vi "Replace_Array_Subset_1D.vi"(7 "E or S RAS":T1, 8 "Subarray RAS":i8[](array[numeric])=[-5, -8], 9 "Element RAS":i8, 10 "Index RAS":i32, 11 "RAS1D":i8[](array[numeric])=[100, -1, -2, 9, 10]) -> (3 "New Array RAS1D":i8[](array[numeric]))   [LabVIEW 2018]
uses:
  Controls/E_S.ctl
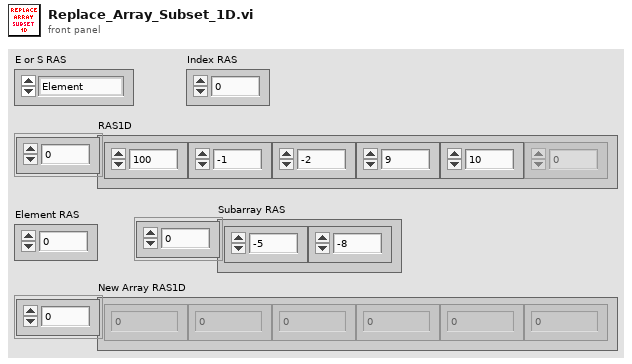
[diagram p1: front panel]
types:
  T1 = typedef "E_S.ctl" = enum16{"Element", "SubArray"}
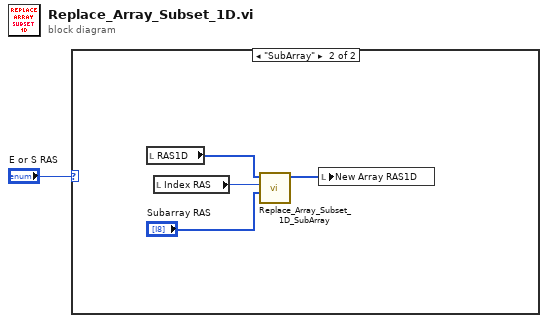
[diagram p0: block diagram]
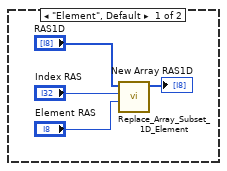
[diagram p2: hidden frame]
diagram:
  n1 = case shown="\"SubArray\"" "E or S RAS" {
    frame "Element", Default {
      n2 = call "Replace_Array_Subset_1D_Element.vi"("Element RAS"="Element RAS", "Index RAS1D"="Index RAS", "RAS1D"="RAS1D") -> ("New Array RAS1D"=→"New Array RAS1D":i8[])  [unwired: 8 in]
    }
    frame "SubArray" {
      n3 = local read "RAS1D"() -> (w8:i8[])
      n4 = local read "Index RAS"() -> (w9:i32)
      n5 = call "Replace_Array_Subset_1D_SubArray.vi"("Subarray RAS1D"="Subarray RAS", "Index RAS1D"=w9, "RAS1D"=w8) -> ("New Array RAS1D"=w6:i8[])  [unwired: 8 in]
      n6 = local write "New Array RAS1D"(w6) -> ()
    }
  }
